vi "Initialize Test Number Generator.vi"(8 "error in (no error)":errorcluster, 11 "niRFSTS Sequence Flow in":refnum<class "niRFSTS Sequence Flow.lvclass">) -> (0 "error out":errorcluster, 3 "niRFSTS Sequence Flow out":refnum<class "niRFSTS Sequence Flow.lvclass">)   [LabVIEW 2018, in "niRFSTS Sequence Flow.lvclass"]
uses:
  niRFSTS Sequence Flow.lvclass
  niRFSTS Sequence Flow.lvclass/niRFSTS Sequence Flow.ctl
  Plugins/Test Number and Bin Generator.lvlibp/Test Number and Bin Generator/Test Number and Bin Generator.lvclass
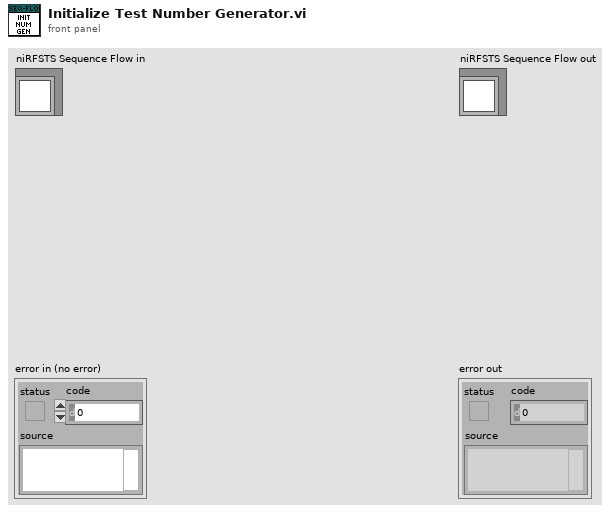
[diagram p1: front panel]
types:
  T1 = typedef "Test Number and Bin Generator.lvlibp/Test Number and Bin Generator.lvclass/Session Handle.ctl" = refnum<data-value>
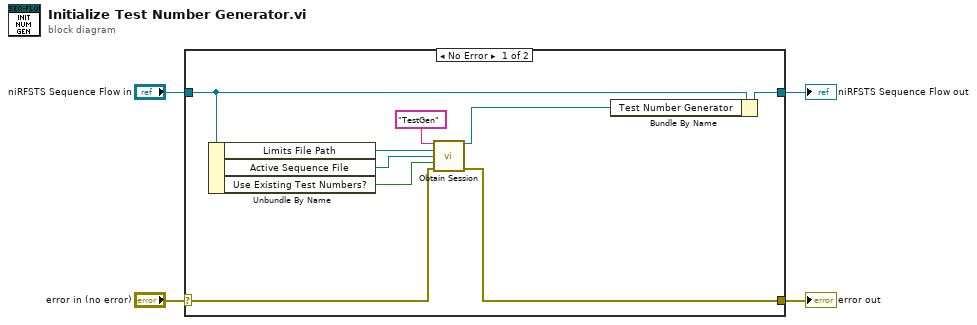
[diagram p0: block diagram]
diagram:
  n1 = case shown="No Error" "error in (no error)" {
    selector: "error in (no error)" -> [w8 w15]
    tunnel: [w7 w15] -> w3
    tunnel: [w6 w14] -> w1
    tunnel: "niRFSTS Sequence Flow in" -> [w12 w14]
    frame No Error {
      n2 = Unbundle By Name(w12) -> ("Limits File Path"=w11:path, "Active Sequence File"=w10:refnum<k7>, "Use Existing Test Numbers?"=w9:bool)
      n3 = call "Obtain Session.vi"("Session  Name ()"="TestGen", "Limits File Path"=w11, "Sequence File"=w10, "Use Existing Test Numbers?"=w9, "error in (no error)"=w8) -> ("Session Handle"=w5:T1, "error out"=w7:errorcluster)  [unwired: 9 in]
      n4 = Bundle By Name(cluster=w12, "Test Number Generator"=w5) -> (w6:refnum<class "niRFSTS Sequence Flow.lvclass">)
    }
    frame Error {
    }
  }
  "error out" <- w3
  "niRFSTS Sequence Flow out" <- w1
